vi "SendTcpCMoveCommand.vi"(6 "機器番号":u8, 8 "SampleName":string="Sample1", 9 "C_Put":string, 10 "CGet":string, 11 "アドレス":string) -> (1 "送信文字列":string, 2 "空?":bool, 3 "Send List Out":cluster{"Address":string, "Data":string}[](array[cluster]))   [LabVIEW 2017]
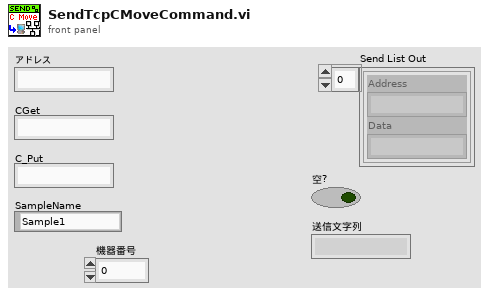
[diagram p1: front panel]
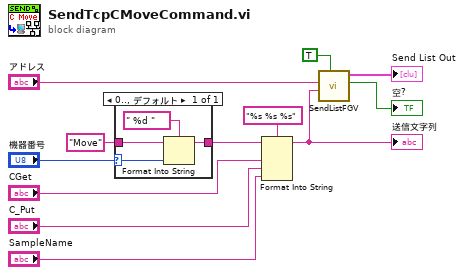
[diagram p0: block diagram]
diagram:
  n1 = case shown="0.., デフォルト" "機器番号" {
    selector: "機器番号" -> [w14]
    tunnel: [w16] -> w2
    tunnel: "Move" ("要素") -> [w13]
    frame 0.., Default {
      n2 = Format Into String(format string=" %d " ("形式文字列"), initial string=w13, w14) -> (resulting string=w16:string)  [unwired: 1 in, 1 out]
    }
  }
  n3 = Format Into String(format string="%s %s %s" ("形式文字列"), initial string=w2, "CGet", "C_Put", "SampleName") -> (resulting string=w1:string)  [unwired: 1 in, 1 out]
  "送信文字列" <- w1
  n4 = call "SendListFGV.vi"("Set"=TRUE, "Data"=w1, "アドレス"="アドレス") -> ("空?"=→"空?":bool, "Send List Out"=→"Send List Out":cluster{"Address":string, "Data":string}[])  [unwired: 6 in, 1 out]
